vi "DriverStation Get Alliance Info.vi"() -> (0 "Replay Number":u16, 1 "Match Number":u16, 2 "Match Type":T3, 3 "Alliance":cluster{"Color":T1, "Position":T2}, 5 "Event Name":string)   [LabVIEW 2026, in "MrcLib.lvlib"]
doc: "Returns the alliance color, field position, and match information as reported by DS or FMS."
uses:
  <menus>/Categories/MRC/MrcLib.lvlib
  <vilib>/Rock Robotics/WPI/DriverStation/WPI_DriverStationAllianceInfo.ctl
  <vilib>/Rock Robotics/WPI/DriverStation/WPI_DriverStationPositionInfo.ctl
  Types/MRC Match TYpe.ctl
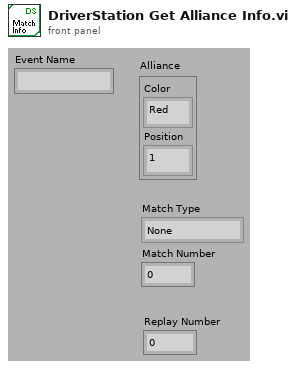
[diagram p1: front panel]
types:
  T1 = typedef "WPI_DriverStationAllianceInfo.ctl" = enum16{"Red", "Blue", "Invalid"}
  T2 = typedef "WPI_DriverStationPositionInfo.ctl" = enum16{"1", "2", "3"}
  T3 = typedef "MrcLib.lvlib/MRC Match TYpe.ctl" = enum32{"None", "Practice", "Qualification", "Elimination"}
  T4 = typedef "MrcLib.lvlib/MRC_ControlData.ctl" = cluster{"controlFlags":u32, "matchTime":u16, "currentOpMode":u64, "gameDataLength":u8, "gameData":cluster{"gameData 0":u8, "gameData 1":u8, "gameData 2":u8, "gameData 3":u8, "gameData 4":u8, "gameData 5":u8, "gameData 6":u8, "gameData 7":u8}}
  T5 = typedef "MRC Str64.ctl" = cluster{"[0]":u8, "[1]":u8, "[2]":u8, "[3]":u8, "[4]":u8, "[5]":u8, "[6]":u8, "[7]":u8, "[8]":u8, "[9]":u8, "[10]":u8, "[11]":u8, "[12]":u8, "[13]":u8, "[14]":u8, "[15]":u8, "[16]":u8, "[17]":u8, "[18]":u8, "[19]":u8, "[20]":u8, "[21]":u8, "[22]":u8, "[23]":u8, "[24]":u8, "[25]":u8, "[26]":u8, "[27]":u8, "[28]":u8, "[29]":u8, "[30]":u8, "[31]":u8, "[32]":u8, "[33]":u8, "[34]":u8, "[35]":u8, "[36]":u8, "[37]":u8, "[38]":u8, "[39]":u8, "[40]":u8, "[41]":u8, "[42]":u8, "[43]":u8, "[44]":u8, "[45]":u8, "[46]":u8, "[47]":u8, "[48]":u8, "[49]":u8, "[50]":u8, "[51]":u8, "[52]":u8, "[53]":u8, "[54]":u8, "[55]":u8, "[56]":u8, "[57]":u8, "[58]":u8, "[59]":u8, "[60]":u8, "[61]":u8, "[62]":u8, "[63]":u8}
  T6 = cluster{"matchNumber":u16, "replayNumber":u8, "matchType":u8, "eventNameLength":u8, "eventName":T5}
  T7 = cluster{"FMSConnected":bool, "SupportOpModes":bool, "Alliance":u32, "RoboWifiMode":bool, "Timed Match":bool}
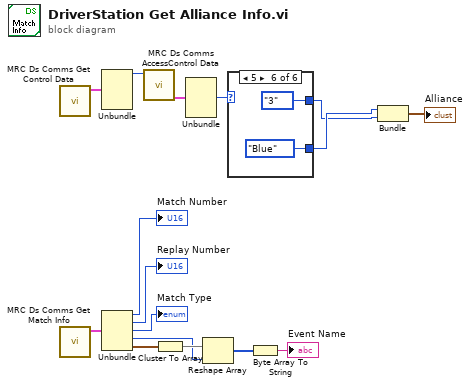
[diagram p0: block diagram]
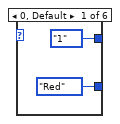
[diagram p2: hidden frame]
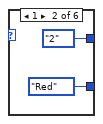
[diagram p3: hidden frame]
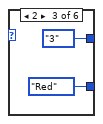
[diagram p4: hidden frame]
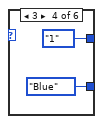
[diagram p5: hidden frame]
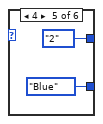
[diagram p6: hidden frame]
diagram:
  n1 = call "MRC Ds Comms Get Control Data.vi"() -> ("data out"=w7:T4)  [unwired: 10 in, 1 out]
  n2 = call "MRC Ds Comms Get Match Info.vi"() -> ("matchInfo out"=w16:T6)  [unwired: 10 in, 1 out]
  n3 = Unbundle(w7) -> ("controlFlags"=w6:u32)  [unwired: 4 out]
  n4 = Unbundle(w16) -> ("matchNumber"=→"Match Number":u16, "replayNumber"=→"Replay Number":u8, "matchType"=→"Match Type":u8, "eventNameLength"=w10:u8, "eventName"=w12:T5)
  n5 = call "MRC Ds Comms AccessControl Data.vi"("controlFlag"=w6) -> ("info"=w5:T7)  [unwired: 7 in, 3 out]
  n6 = Cluster To Array(cluster=w12) -> (array=w11:u8[])
  n7 = Unbundle(w5) -> ("Alliance"=w4:u32)  [unwired: 4 out]
  n8 = Reshape Array(w11, w10) -> (w9:u8[])
  n9 = case shown="5" w4 {
    tunnel: [WPI_DriverStationAllianceInfo."Red" ("Alliance") WPI_DriverStationAllianceInfo."Red" ("Alliance") WPI_DriverStationAllianceInfo."Red" ("Alliance") WPI_DriverStationAllianceInfo."Blue" ("Alliance") WPI_DriverStationAllianceInfo."Blue" ("Alliance") WPI_DriverStationAllianceInfo."Blue" ("Alliance")] -> w3
    tunnel: [WPI_DriverStationPositionInfo."1" ("Position") WPI_DriverStationPositionInfo."2" ("Position") WPI_DriverStationPositionInfo."3" ("Position") WPI_DriverStationPositionInfo."1" ("Position") WPI_DriverStationPositionInfo."2" ("Position") WPI_DriverStationPositionInfo."3" ("Position")] -> w2
    frame 0, Default {
    }
    frame 1 {
    }
    frame 2 {
    }
    frame 3 {
    }
    frame 4 {
    }
    frame 5 {
    }
  }
  n10 = Byte Array To String(unsigned byte array=w9) -> (string=→"Event Name":string)
  n11 = Bundle("Alliance"=w3, "Position"=w2) -> (→"Alliance":cluster{"Alliance":T1, "Position":T2})  [unwired: 1 in]
